vi "FPGA counter.vi"(1 "no reset?":bool) -> (0 "count":u8)   [LabVIEW 2010]
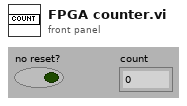
[diagram p1: front panel]
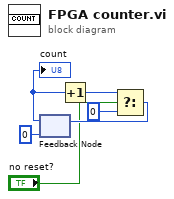
[diagram p0: block diagram]
diagram:
  n1 = feedback #1(u8 0 ("y")) -> (w5:u8)
  "count" <- w5
  n2 = Increment(x=w5) -> (x+1=w4:u8)
  n3 = Select(t=w4, s="no reset?", f=u8 0) -> (s? t:f=w3:u8)
  n4 = feedback-in #1(w3) -> ()
